vi "Replay Data from History.vi"(8 "error in (no error)":errorcluster, 10 "Data in":string[](array[string]), 11 "Data in":T1={"Class"={"Ants"=refnum, "Layer"=refnum, "Templates"=refnum, "Icon"=refnum, "Glyph"=refnum, "Settings"=refnum, "Tools"=refnum}, "Ref"={"Add Layer"=refnum, "Remove Layer"=refnum, "Line Text"=[], "Body Text Spec"=refnum, "DNL_Font"=refnum, "glyph path str"=refnum, "templates path str"=refnum, "Arrow Up"=refnum, "Arrow Down"=refnum, "IE VI Ref"=refnum, "Glyphs tree"=refnum, "Templates tree"=refnum, "Layer Icon Text"=refnum, "Layer Template"=refnum, "Body Text"=refnum, "Search Templates"=refnum, "TextMarker"=refnum, "Tab Control"=refnum, "Search Glyphs"=refnum, "Line Color"=refnum, "DNL_Glyphs []"=refnum, "Fill Color"=refnum, "Tools"=refnum, "Icon"=refnum, "Preview"=refnum, "Ants"=refnum, "Terminals"=refnum, "menu reference"=refnum, "LayerNames"=[], "GlyphLoadAnimation"=refnum, "TemplateLoadAnimation"=refnum, "refreshGlyphs"=refnum, "refreshTemplates"=refnum}, "Support"={"AntsRect"={"left"=0, "top"=0, "right"=0, "bottom"=0}, "Mouse Move Coords"={"Horizontal"=0, "Vertical"=0}, "Mouse Down Coords"={"Horizontal"=0, "Vertical"=0}, "Temp Coord"={"Horizontal"=0, "Vertical"=0}, "Action"=enum."Default", "Edge Color"=4914962, "Fill Color"=16860, "Mouse Down?"=FALSE, "Draft Mode?"=FALSE, "Temp Icon"=bytes[3102], "CTRL Pressed"=FALSE, "Move Selection?"=FALSE, "AntsRect Orig"={"left"=0, "top"=0, "right"=0, "bottom"=0}, "Text"="", "TM Set?"=FALSE, "Mouse inside icon?"=FALSE, "Tool (old value)"=0, "Pencil Move Color"=0, "Swap Colors?"=FALSE, "Shift pressed?"=FALSE}}) -> (0 "error out":errorcluster, 3 "Data out":T1={"Class"={"Ants"=refnum, "Layer"=refnum, "Templates"=refnum, "Icon"=refnum, "Glyph"=refnum, "Settings"=refnum, "Tools"=refnum}, "Ref"={"Add Layer"=refnum, "Remove Layer"=refnum, "Line Text"=[], "Body Text Spec"=refnum, "DNL_Font"=refnum, "glyph path str"=refnum, "templates path str"=refnum, "Arrow Up"=refnum, "Arrow Down"=refnum, "IE VI Ref"=refnum, "Glyphs tree"=refnum, "Templates tree"=refnum, "Layer Icon Text"=refnum, "Layer Template"=refnum, "Body Text"=refnum, "Search Templates"=refnum, "TextMarker"=refnum, "Tab Control"=refnum, "Search Glyphs"=refnum, "Line Color"=refnum, "DNL_Glyphs []"=refnum, "Fill Color"=refnum, "Tools"=refnum, "Icon"=refnum, "Preview"=refnum, "Ants"=refnum, "Terminals"=refnum, "menu reference"=refnum, "LayerNames"=[], "GlyphLoadAnimation"=refnum, "TemplateLoadAnimation"=refnum, "refreshGlyphs"=refnum, "refreshTemplates"=refnum}, "Support"={"AntsRect"={"left"=0, "top"=0, "right"=0, "bottom"=0}, "Mouse Move Coords"={"Horizontal"=0, "Vertical"=0}, "Mouse Down Coords"={"Horizontal"=0, "Vertical"=0}, "Temp Coord"={"Horizontal"=0, "Vertical"=0}, "Action"=enum."Default", "Edge Color"=4914962, "Fill Color"=16860, "Mouse Down?"=FALSE, "Draft Mode?"=FALSE, "Temp Icon"=bytes[3102], "CTRL Pressed"=FALSE, "Move Selection?"=FALSE, "AntsRect Orig"={"left"=0, "top"=0, "right"=0, "bottom"=0}, "Text"="", "TM Set?"=FALSE, "Mouse inside icon?"=FALSE, "Tool (old value)"=0, "Pencil Move Color"=0, "Swap Colors?"=FALSE, "Shift pressed?"=FALSE}})   [LabVIEW 2020, in "lv_icon.lvlib" / "History.lvclass"]
uses:
  History.lvclass
  Class/Ants/Ants.lvclass
  Class/FakedArray/FakedArray.lvclass
  vi.lib/LabVIEW Icon API/lv_icon/Classes/Icon/Icon.lvclass
  Class/Icon Library/Glyph.lvclass
  Class/Settings/Settings.lvclass
  Class/Tools/Tools Paint.lvclass
  History.lvclass/History.ctl
  vi.lib/LabVIEW Icon API/lv_icon/Controls/Layer.ctl
  vi.lib/LabVIEW Icon API/lv_icon/Controls/Graphic.ctl
  vi.lib/LabVIEW Icon API/lv_icon/Controls/BodyText.ctl
  vi.lib/LabVIEW Icon API/lv_icon/Controls/Font.ctl
  vi.lib/LabVIEW Icon API/lv_icon/Controls/Alignment.ctl
  <vilib>/Utility/miscctls.llb/LVPoint32TypeDef.ctl
  Controls/SupportClass_Action.ctl
  vi.lib/LabVIEW Icon API/lv_icon/Controls/IEColor.ctl
  Controls/SupportClass.ctl
  Controls/References Cluster.ctl
  lv_icon.lvlib
  Controls/IE Classes.ctl
  Controls/Global Data.ctl
panel:
  in  "Body Text 2":T8={"Line 1 text"="", "Line 2 text"="", "Line 3 text"="", "Line 4 text"="", "Line 1 color"=0, "Line 2 color"=0, "Line 3 color"=0, "Line 4 color"=0, "Body Text Spec"={"Font"="", "Alignment"=0, "Size"=3}, "Center text vertically"=FALSE, "Capitalize Text"=FALSE} {"Body Text Spec"."Alignment" items=["left", "center", "right"]}
  in  "?":T11
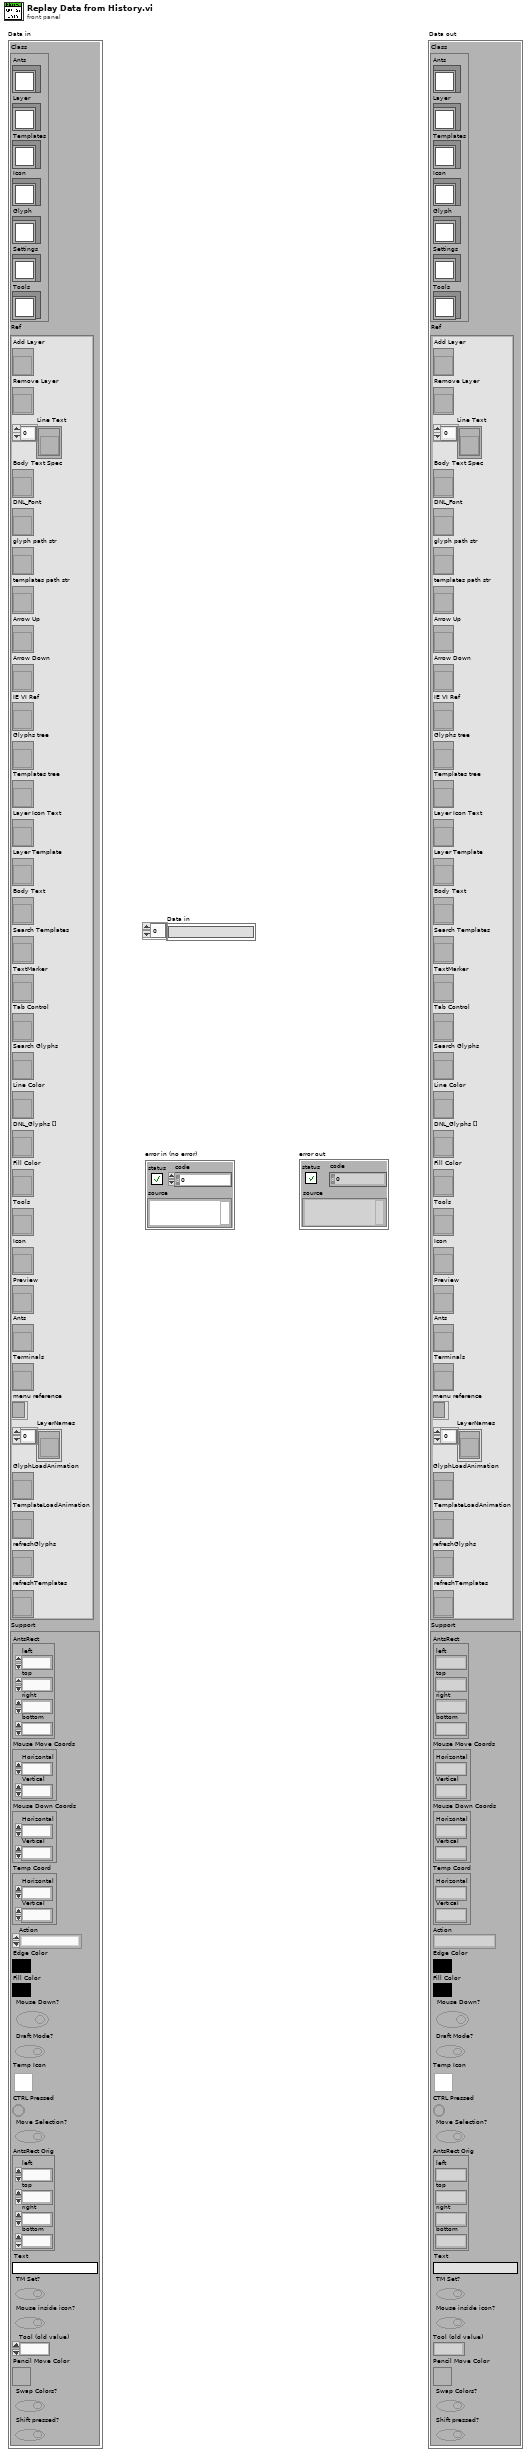
[diagram p1: front panel]
types:
  T1 = typedef "lv_icon.lvlib/Global Data.ctl" = cluster{"Class":T2, "Ref":T3, "Support":T4}
  T2 = typedef "IE Classes.ctl" = cluster{"Ants":refnum<class "Ants.lvclass">, "Layer":refnum<class "FakedArray.lvclass">, "Templates":refnum<class "FakedArray.lvclass">, "Icon":refnum<class "Icon.lvclass">, "Glyph":refnum<class "Glyph.lvclass">, "Settings":refnum<class "Settings.lvclass">, "Tools":refnum<class "Tools Paint.lvclass">}
  T3 = typedef "lv_icon.lvlib/References Cluster.ctl" = cluster{"Add Layer":refnum<vi>, "Remove Layer":refnum<vi>, "Line Text":refnum<vi>[], "Body Text Spec":refnum<vi>, "DNL_Font":refnum<vi>, "glyph path str":refnum<vi>, "templates path str":refnum<vi>, "Arrow Up":refnum<vi>, "Arrow Down":refnum<vi>, "IE VI Ref":refnum<vi>, "Glyphs tree":refnum<vi>, "Templates tree":refnum<vi>, "Layer Icon Text":refnum<vi>, "Layer Template":refnum<vi>, "Body Text":refnum<vi>, "Search Templates":refnum<vi>, "TextMarker":refnum<vi>, "Tab Control":refnum<vi>, "Search Glyphs":refnum<vi>, "Line Color":refnum<vi>, "DNL_Glyphs []":refnum<vi>, "Fill Color":refnum<vi>, "Tools":refnum<vi>, "Icon":refnum<vi>, "Preview":refnum<vi>, "Ants":refnum<vi>, "Terminals":refnum<vi>, "menu reference":refnum<k9>, "LayerNames":refnum<vi>[], "GlyphLoadAnimation":refnum<vi>, "TemplateLoadAnimation":refnum<vi>, "refreshGlyphs":refnum<vi>, "refreshTemplates":refnum<vi>}
  T4 = typedef "SupportClass.ctl" = cluster{"AntsRect":cluster{"left":i16, "top":i16, "right":i16, "bottom":i16}, "Mouse Move Coords":T5, "Mouse Down Coords":T5, "Temp Coord":T5, "Action":T6, "Edge Color":T7, "Fill Color":T7, "Mouse Down?":bool, "Draft Mode?":bool, "Temp Icon":picture, "CTRL Pressed":bool, "Move Selection?":bool, "AntsRect Orig":cluster{"left":i16, "top":i16, "right":i16, "bottom":i16}, "Text":string, "TM Set?":bool, "Mouse inside icon?":bool, "Tool (old value)":u32, "Pencil Move Color":u32, "Swap Colors?":bool, "Shift pressed?":bool}
  T5 = typedef "LVPoint32TypeDef.ctl" = cluster{"Horizontal":i32, "Vertical":i32}
  T6 = typedef "SupportClass_Action.ctl" = enum16{"Default", "Move Selection", "Glyph Library", "Tool"}
  T7 = typedef "IEColor.ctl" = u32
  T8 = typedef "BodyText.ctl" = cluster{"Line 1 text":string, "Line 2 text":string, "Line 3 text":string, "Line 4 text":string, "Line 1 color":u32, "Line 2 color":u32, "Line 3 color":u32, "Line 4 color":u32, "Body Text Spec":cluster{"Font":T9, "Alignment":T10, "Size":u8}, "Center text vertically":bool, "Capitalize Text":bool}
  T9 = typedef "Font.ctl" = string
  T10 = typedef "Alignment.ctl" = u16
  T11 = typedef "Graphic.ctl" = cluster{"Rectangle":cluster{"left":i16, "top":i16, "right":i16, "bottom":i16}, "Path":path, "Image":picture, "Filter":string, "FileName":string}
  T12 = typedef "Layer.ctl" = cluster{"LayerIcon":picture, "LayerName":string, "Opacity":u8, "Visibility?":bool}
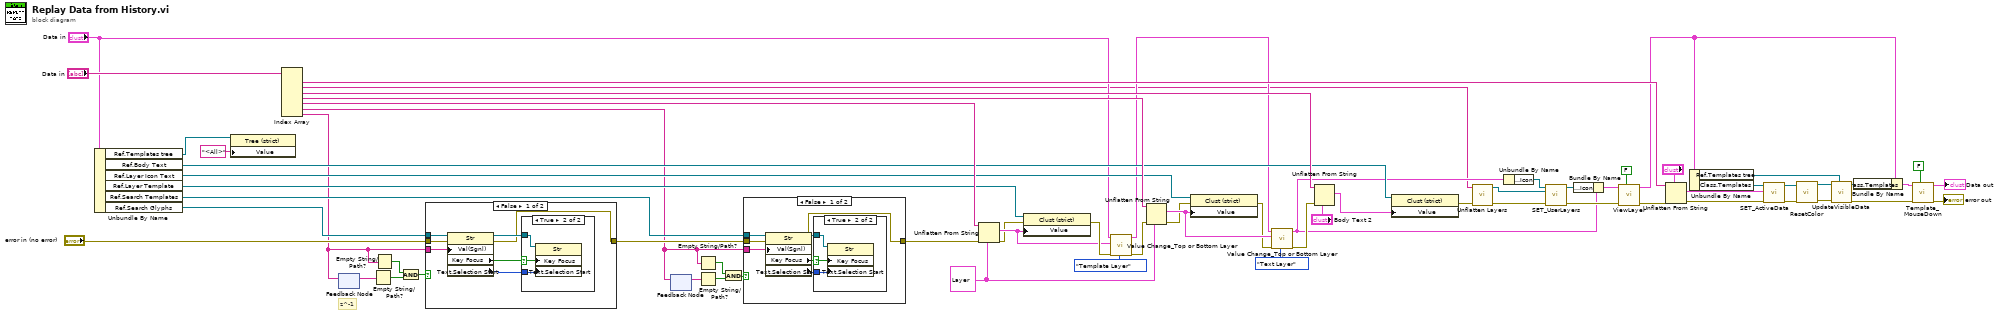
[diagram p0: block diagram]
diagram:
  w49 = T12 {"LayerIcon"=bytes[3102], "LayerName"="", "Opacity"=100, "Visibility?"=TRUE}
  # "z^-1"
  n1 = Unbundle By Name("Data in") -> ("Ref.Templates tree"=w39:refnum<vi>, "Ref.Body Text"=w51:refnum<vi>, "Ref.Layer Icon Text"=w52:refnum<vi>, "Ref.Layer Template"=w53:refnum<vi>, "Ref.Search Templates"=w13:refnum<vi>, "Ref.Search Glyphs"=w15:refnum<vi>)
  n2 = property class="Tree (strict)"(reference=w39, "Value"="<All>") -> ()  [unwired: 1 in, 2 out]
  n3 = Index Array(array="Data in") -> (element #1=w56:string, element #2=w16:string, element #3=w65:string, element #4=w66:string, element #5=w67:string, element #6=w3:string, element #7=w7:string)  [unwired: 7 in]
  n4 = feedback-in #1(w7) -> ()
  n5 = feedback #1() -> (w8:string)  [unwired: 1 in]
  n6 = Empty String/Path?(string/path=w8) -> (empty?=w10:bool)
  n7 = Empty String/Path?(string/path=w7) -> (empty?=w5:bool)
  n8 = And(x=w5, y=w10) -> (x .and. y?=w6:bool)
  n9 = case shown="False" w6 {
    tunnel: w7 -> [w74 _]
    tunnel: w15 -> [w73 _]
    tunnel: "error in (no error)" -> [w72 w78]
    tunnel: [w68 w78] -> w12
    frame False {
      n10 = property class="Str"(reference=w73, error in=w72, "Val(Sgnl)"=w74) -> (reference out=w69:refnum<vi>, error out=w68:errorcluster, "Key Focus"=w71:bool, "Text.Selection Start"=w70:u32)
      n11 = case shown="True" w71 {
        selector: w71 -> [_ w76]
        tunnel: w70 -> [_ w77]
        tunnel: w69 -> [_ w75]
        frame False {
        }
        frame True {
          n12 = property class="Str"(reference=w75, "Key Focus"=w76, "Text.Selection Start"=w77) -> ()  [unwired: 1 in, 2 out]
        }
      }
    }
    frame True {
    }
  }
  n13 = feedback #2() -> (w4:string)  [unwired: 1 in]
  n14 = feedback-in #2(w3) -> ()
  n15 = Empty String/Path?(string/path=w3) -> (empty?=w1:bool)
  n16 = Empty String/Path?(string/path=w4) -> (empty?=w9:bool)
  n17 = And(x=w1, y=w9) -> (x .and. y?=w2:bool)
  n18 = case shown="False" w2 {
    tunnel: w13 -> [w82 _]
    tunnel: w12 -> [w81 w89]
    tunnel: w3 -> [w80 _]
    tunnel: [w79 w89] -> w11
    frame False {
      n19 = property class="Str"(reference=w82, error in=w81, "Val(Sgnl)"=w80) -> (reference out=w85:refnum<vi>, error out=w79:errorcluster, "Key Focus"=w83:bool, "Text.Selection Start"=w84:u32)
      n20 = case shown="True" w83 {
        selector: w83 -> [_ w87]
        tunnel: w84 -> [_ w88]
        tunnel: w85 -> [_ w86]
        frame False {
        }
        frame True {
          n21 = property class="Str"(reference=w86, "Key Focus"=w87, "Text.Selection Start"=w88) -> ()  [unwired: 1 in, 2 out]
        }
      }
    }
    frame True {
    }
  }
  n22 = Unflatten From String(type=w49, binary string=w67, error in (no error)=w11) -> (value=w45:T12, error out=w35:errorcluster)  [unwired: 3 out]
  n23 = property class="Clust (strict)"(reference=w53, error in=w35, "Value"=w45) -> (error out=w46:errorcluster)  [unwired: 1 out]
  n24 = call "Value Change_Top or Bottom Layer.vi"("Type"=enum16{"Template Layer", "Text Layer"}."Template Layer", "error in (no error)"=w46, "Data"=w45, "Data in"="Data in") -> ("error out"=w37:errorcluster, "Data out"=w23:T1)  [unwired: 6 out]
  n25 = Unflatten From String(type=w49, binary string=w66, error in (no error)=w37) -> (value=w43:T12, error out=w36:errorcluster)  [unwired: 3 out]
  n26 = property class="Clust (strict)"(reference=w52, error in=w36, "Value"=w43) -> (error out=w42:errorcluster)  [unwired: 1 out]
  n27 = call "Value Change_Top or Bottom Layer.vi"("Type"=enum16{"Template Layer", "Text Layer"}."Text Layer", "error in (no error)"=w42, "Data"=w43, "Data in"=w23) -> ("error out"=w41:errorcluster, "Data out"=w20:T1)  [unwired: 6 out]
  n28 = Unflatten From String(type="Body Text 2", binary string=w65, error in (no error)=w41) -> (value=w63:T8)  [unwired: 1 in, 3 out]
  n29 = property class="Clust (strict)"(reference=w51, "Value"=w63) -> (error out=w19:errorcluster)  [unwired: 1 in, 1 out]
  n30 = call "Unflatten Layers.vi"("Error In"=w19, "String"=w16) -> ("Error Out"=w18:errorcluster, "Layers"=w17:refnum<class "Layer.lvclass">[])  [unwired: 8 in]
  n31 = Unbundle By Name(w20) -> ("Class.Icon"=w34:refnum<class "Icon.lvclass">)
  n32 = call-dynamic "SET_UserLayers.vi"("error in (no error)"=w18, "Layers"=w17, "Icon.lvclass in"=w34) -> ("error out"=w26:errorcluster, "Icon.lvclass out"=w33:refnum<class "Icon.lvclass">)  [unwired: 7 in]
  n33 = Bundle By Name(cluster=w20, "Class.Icon"=w33) -> (w32:T1)
  n34 = call "ViewLayer.vi"("Add to Undo?"=FALSE, "error in (no error)"=w26, "Data in"=w32) -> ("error out"=w50:errorcluster, "Data out"=w21:T1)  [unwired: 1 in, 6 out]
  n35 = Unflatten From String(type="?", binary string=w56, error in (no error)=w50) -> (value=w61:T11, error out=w31:errorcluster)  [unwired: 3 out]
  n36 = Unbundle By Name(w21) -> ("Ref.Templates tree"=w22:refnum<vi>, "Class.Templates"=w30:refnum<class "FakedArray.lvclass">)
  n37 = call-dynamic "SET_ActiveData.vi"("error in (no error)"=w31, "Active Data"=w61, "FakedArray.lvclass in"=w30) -> ("error out"=w58:errorcluster, "FakedArray.lvclass out"=w57:refnum<class "FakedArray.lvclass">)  [unwired: 7 out]
  n38 = call "ResetColor.vi"("error in (no error)"=w58, "FakedArray in"=w57) -> ("error out"=w60:errorcluster, "FakedArray out"=w59:refnum<class "FakedArray.lvclass">)  [unwired: 8 out]
  n39 = call-dynamic "UpdateVisibleData.vi"("Templates tree"=w22, "error in (no error)"=w60, "FakedArray in"=w59) -> ("error out"=w25:errorcluster, "FakedArray out"=w29:refnum<class "FakedArray.lvclass">)  [unwired: 2 in, 5 out]
  n40 = Bundle By Name(cluster=w21, "Class.Templates"=w29) -> (w28:T1)
  n41 = call "Template_MouseDown.vi"("Add to Undo?"=FALSE, "error in"=w25, "Data in"=w28) -> ("error out"=→"error out":errorcluster, "Data out"=→"Data out":T1)  [unwired: 2 in, 5 out]
